vi "create_AVS_Data_header.vi"() -> (3 "String":string)   [LabVIEW 2019]
uses:
  Instrument_Setup.vi
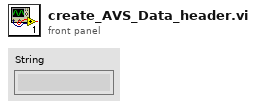
[diagram p1: front panel]
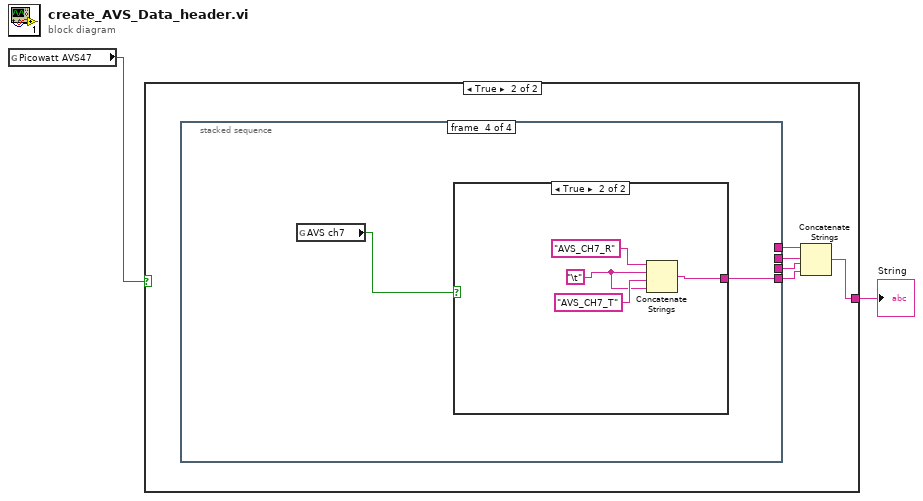
[diagram p0: block diagram]
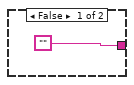
[diagram p2: hidden frame]
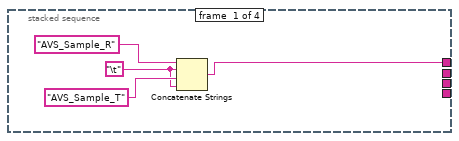
[diagram p3: hidden frame]
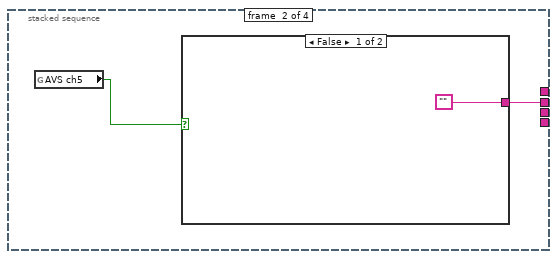
[diagram p4: hidden frame]
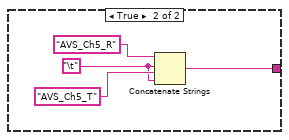
[diagram p5: hidden frame]
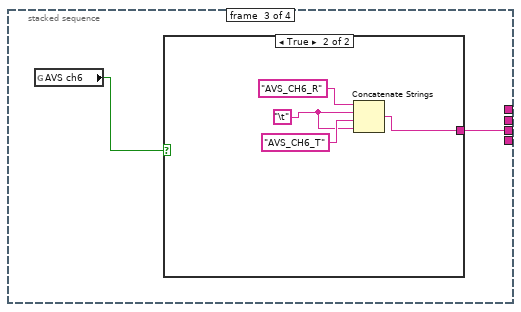
[diagram p6: hidden frame]
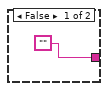
[diagram p7: hidden frame]
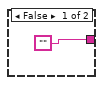
[diagram p8: hidden frame]
diagram:
  n1 = global read "Instrument_Setup.vi" "Picowatt AVS47"() -> (w2:bool)
  n2 = case shown="True" w2 {
    tunnel: ["" w7] -> w1
    frame False {
    }
    frame True {
      n3 = stacked-sequence {
        tunnel: [w9 _ _ _] -> w8
        tunnel: [_ w13 _ _] -> w6
        tunnel: [_ _ w20 _] -> w5
        tunnel: [_ _ _ w27] -> w4
        frame #0 {
          w10 = "\t"
          n4 = Concatenate Strings("AVS_Sample_R", w10, "AVS_Sample_T", w10) -> (w9:string)
        }
        frame #1 {
          n5 = global read "Instrument_Setup.vi" "AVS ch5"() -> (w14:bool)
          n6 = case shown="False" w14 {
            tunnel: ["" w16] -> w13
            frame False {
            }
            frame True {
              w17 = "\t"
              n7 = Concatenate Strings("AVS_Ch5_R", w17, "AVS_Ch5_T", w17) -> (w16:string)
            }
          }
        }
        frame #2 {
          n8 = global read "Instrument_Setup.vi" "AVS ch6"() -> (w21:bool)
          n9 = case shown="True" w21 {
            tunnel: ["" w23] -> w20
            frame False {
            }
            frame True {
              w24 = "\t"
              n10 = Concatenate Strings("AVS_CH6_R", w24, "AVS_CH6_T", w24) -> (w23:string)
            }
          }
        }
        frame #3 {
          n11 = global read "Instrument_Setup.vi" "AVS ch7"() -> (w28:bool)
          n12 = case shown="True" w28 {
            tunnel: ["" w30] -> w27
            frame False {
            }
            frame True {
              w31 = "\t"
              n13 = Concatenate Strings("AVS_CH7_R", w31, "AVS_CH7_T", w31) -> (w30:string)
            }
          }
        }
      }
      n14 = Concatenate Strings(w8, w6, w5, w4) -> (w7:string)
    }
  }
  "String" <- w1
